vi "basic_calculator.vi"() -> ()   [LabVIEW 2022 SP3]
panel:
  in  "stop":bool
  out "String":string
  in  "Cluster":T1
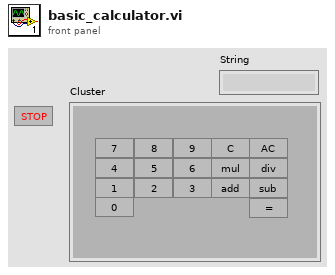
[diagram p1: front panel]
types:
  T1 = cluster{"7":bool, "4":bool, "9":bool, "5":bool, "6":bool, "1":bool, "2":bool, "3":bool, "0":bool, "AC":bool, "C":bool, "add":bool, "sub":bool, "mul":bool, "8":bool, "div":bool, "=":bool}
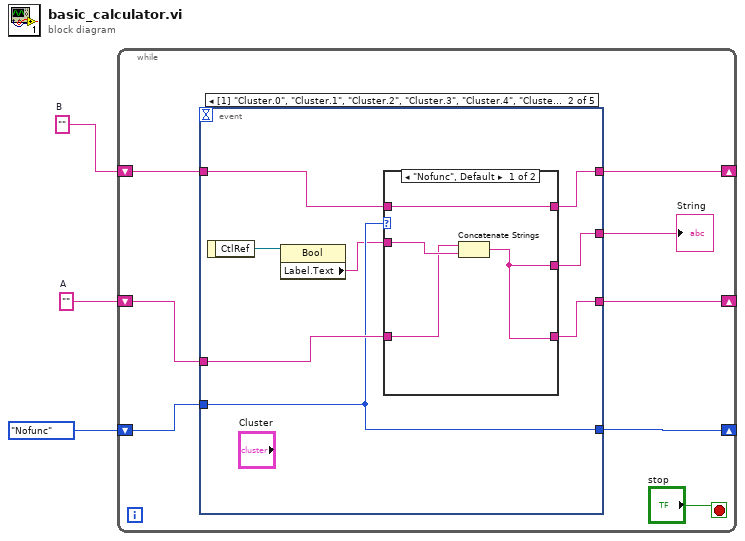
[diagram p0: block diagram]
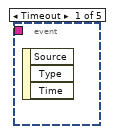
[diagram p2: hidden frame]
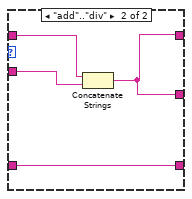
[diagram p3: hidden frame]
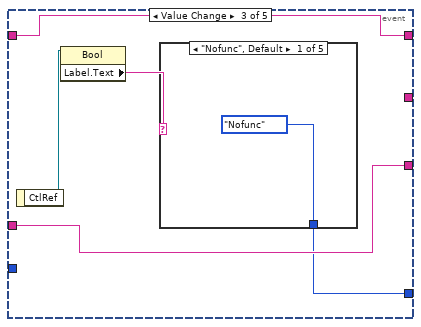
[diagram p4: hidden frame]
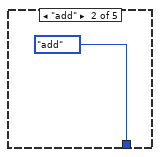
[diagram p5: hidden frame]
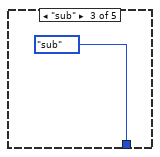
[diagram p6: hidden frame]
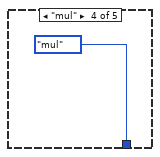
[diagram p7: hidden frame]
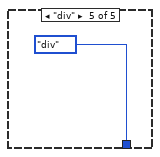
[diagram p8: hidden frame]
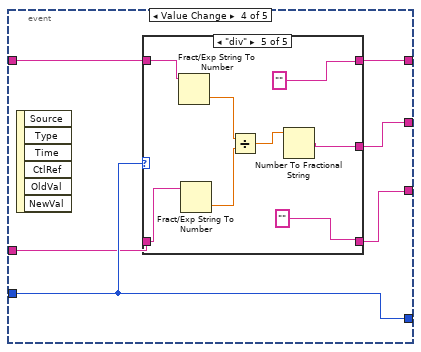
[diagram p9: hidden frame]
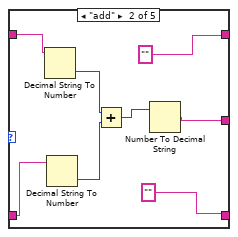
[diagram p11: hidden frame]
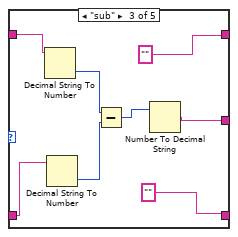
[diagram p12: hidden frame]
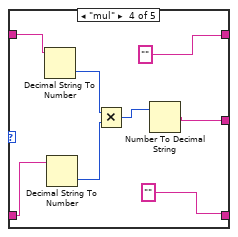
[diagram p13: hidden frame]
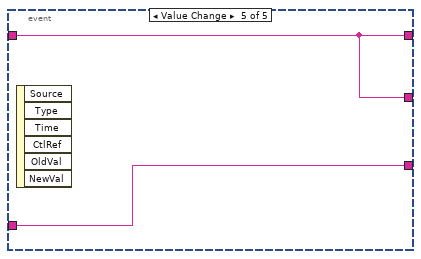
[diagram p14: hidden frame]
diagram:
  w2 = ""  # A
  w3 = ""  # B
  n1 = while {
    shift-right: [w8] -> _
    shift-left: w3 -> [w10]
    shift-right: [w7] -> _
    shift-left: w2 -> [w11]
    shift-right: [w6] -> _
    shift-left: enum16{"", "Nofunc", "add", "sub", "mul", "div"}."Nofunc" -> [w9]
    stop <- "stop" stop-if-true
    n2 = event shown="[1] \"Cluster.0\", \"Cluster.1\", \"Cluster.2\", \"Cluster.3\", \"Cluster.4\", \"Cluster.5\", \"Cluster.6\", \"Cluster.7\", \"Cluster.8\", \"Cluster.9\": Value Change" {
      selector: _ -> [_ _ _ _ _]
      dyn-events: _ -> [_ _ _ _ _]
      timeout: _ -> [_ _ _ _ _]
      tunnel: w11 -> [_ w17 w31 w40 w78]
      tunnel: w10 -> [_ w18 w30 w42 w79]
      tunnel: w9 -> [_ w16 _ w43 _]
      tunnel: [_ w15 w30 w41 w79] -> w8
      tunnel: [_ w14 w31 w39 w78] -> w7
      tunnel: [_ w16 w28 w43 _] -> w6
      tunnel: [_ w13 _ w38 w79] -> w5
      event Timeout {
        n3 = event-data() -> ()  [unwired: 1 in, 3 out]
      }
      event "Cluster.0", "Cluster.1", "Cluster.2", "Cluster.3", "Cluster.4", "Cluster.5", "Cluster.6", "Cluster.7", "Cluster.8", "Cluster.9": Value Change {
        n4 = event-data() -> ("CtlRef"=w19:refnum<vi>)  [unwired: 1 in]
        n5 = property class="Bool"(reference=w19) -> ("Label.Text"=w12:string)  [unwired: 1 in, 2 out]
        n6 = case shown="\"Nofunc\", Default" w16 {
          tunnel: w18 -> [w21 w26]
          tunnel: w17 -> [w22 w25]
          tunnel: [w21 w24] -> w15
          tunnel: [w20 w25] -> w14
          tunnel: [w20 w24] -> w13
          tunnel: w12 -> [w23 w27]
          frame "Nofunc", Default {
            n7 = Concatenate Strings(w22, w23) -> (w20:string)
          }
          frame "add".."div" {
            n8 = Concatenate Strings(w26, w27) -> (w24:string)
          }
        }
      }
      event "Cluster.add", "Cluster.sub", "Cluster.mul", "Cluster.div": Value Change {
        n9 = event-data() -> ("CtlRef"=w29:refnum<vi>)  [unwired: 1 in]
        n10 = property class="Bool"(reference=w29) -> ("Label.Text"=w32:string)  [unwired: 1 in, 2 out]
        n11 = case shown="\"Nofunc\", Default" w32 {
          tunnel: [enum16{"", "Nofunc", "add", "sub", "mul", "div"}."Nofunc" enum16{"", "Nofunc", "add", "sub", "mul", "div"}."add" enum16{"", "Nofunc", "add", "sub", "mul", "div"}."sub" enum16{"", "Nofunc", "add", "sub", "mul", "div"}."mul" enum16{"", "Nofunc", "add", "sub", "mul", "div"}."div"] -> w28
          frame "Nofunc", Default {
          }
          frame "add" {
          }
          frame "sub" {
          }
          frame "mul" {
          }
          frame "div" {
          }
        }
      }
      event "Cluster.=": Value Change {
        n12 = event-data() -> ()  [unwired: 1 in, 6 out]
        n13 = case shown="\"div\"" w43 {
          tunnel: w42 -> [w44 w53 w61 w69 w77]
          tunnel: [w44 "" "" "" ""] -> w41
          tunnel: w40 -> [w45 w52 w60 w68 w76]
          tunnel: [w45 "" "" "" ""] -> w39
          tunnel: [w44 w48 w56 w64 w72] -> w38
          frame "Nofunc", Default {
          }
          frame "add" {
            n14 = Decimal String To Number(string=w53) -> (number=w50:i32)  [unwired: 2 in, 1 out]
            n15 = Decimal String To Number(string=w52) -> (number=w51:i32)  [unwired: 2 in, 1 out]
            n16 = Add(x=w50, y=w51) -> (x+y=w49:i32)
            n17 = Number To Decimal String(number=w49) -> (decimal integer string=w48:string)  [unwired: 1 in]
          }
          frame "sub" {
            n18 = Decimal String To Number(string=w61) -> (number=w58:i32)  [unwired: 2 in, 1 out]
            n19 = Decimal String To Number(string=w60) -> (number=w59:i32)  [unwired: 2 in, 1 out]
            n20 = Subtract(x=w58, y=w59) -> (x-y=w57:i32)
            n21 = Number To Decimal String(number=w57) -> (decimal integer string=w56:string)  [unwired: 1 in]
          }
          frame "mul" {
            n22 = Decimal String To Number(string=w69) -> (number=w66:i32)  [unwired: 2 in, 1 out]
            n23 = Decimal String To Number(string=w68) -> (number=w67:i32)  [unwired: 2 in, 1 out]
            n24 = Multiply(x=w66, y=w67) -> (x*y=w65:i32)
            n25 = Number To Decimal String(number=w65) -> (decimal integer string=w64:string)  [unwired: 1 in]
          }
          frame "div" {
            n26 = Fract/Exp String To Number(string=w77) -> (number=w74:dbl)  [unwired: 3 in, 1 out]
            n27 = Fract/Exp String To Number(string=w76) -> (number=w75:dbl)  [unwired: 3 in, 1 out]
            n28 = Divide(x=w74, y=w75) -> (x/y=w73:dbl)
            n29 = Number To Fractional String(number=w73) -> (F-format string=w72:string)  [unwired: 3 in]
          }
        }
      }
      event "Cluster.C": Value Change {
        n30 = event-data() -> ()  [unwired: 1 in, 6 out]
      }
    }
    "String" <- w5
  }
